vi "Get Active Project Details.vi"(8 "error in":errorcluster) -> (0 "error out":errorcluster, 2 "name":string, 3 "path":path)   [LabVIEW 2021, in "Create Measurement Plug-In Client.lvlib"]
uses:
  Create Measurement Plug-In Client.lvlib
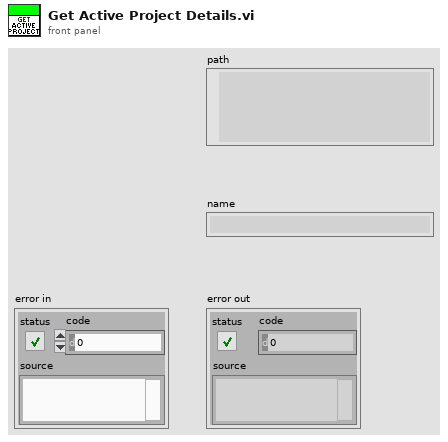
[diagram p1: front panel]
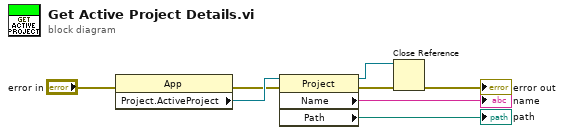
[diagram p0: block diagram]
diagram:
  n1 = property class="App"(error in="error in") -> (error out=w6:errorcluster, "Project.ActiveProject"=w7:refnum<vi>)  [unwired: 1 in, 1 out]
  n2 = property class="Project"(reference=w7, error in=w6) -> (reference out=w1:refnum<vi>, error out=w5:errorcluster, "Name"=→"name":string, "Path"=→"path":path)
  n3 = Close Reference(reference=w1, error in (no error)=w5) -> (error out=→"error out":errorcluster)
